vi "OpenURI.vi"   [LabVIEW 2020]
uses:
  <vilib>/LabVIEW Open Source Project/OpenURI/uri/URI.lvclass
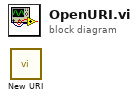
[diagram p0: block diagram]
diagram:
  n1 = call <vilib>:"New URI.vi"() -> ()  [unwired: 10 in, 2 out]
